vi "testAssertConnectorPanesMatchExpectedMissingFails.vi"(8 "error in (no error)":errorcluster, 11 "TestCase in":refnum<class "VeriStandTestCaseUnitTests.lvclass">) -> (0 "error out":errorcluster, 3 "TestCase out":refnum<class "VeriStandTestCaseUnitTests.lvclass">)   [LabVIEW 2015, in "VeriStandTestCaseUnitTests.lvclass"]
uses:
  VeriStandTestCaseUnitTests.lvclass
  <userlib>/_OpenG.lib/file/file.llb/Build Path - File Names Array - path__ogtk.vi
  <vilib>/addons/_JKI Toolkits/VI Tester/TestCase.llb/TestCase.lvclass
  VeriStandTestCase.lvclass
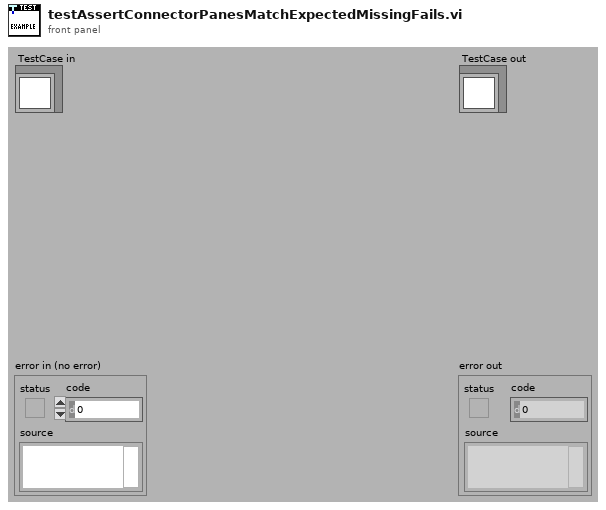
[diagram p1: front panel]
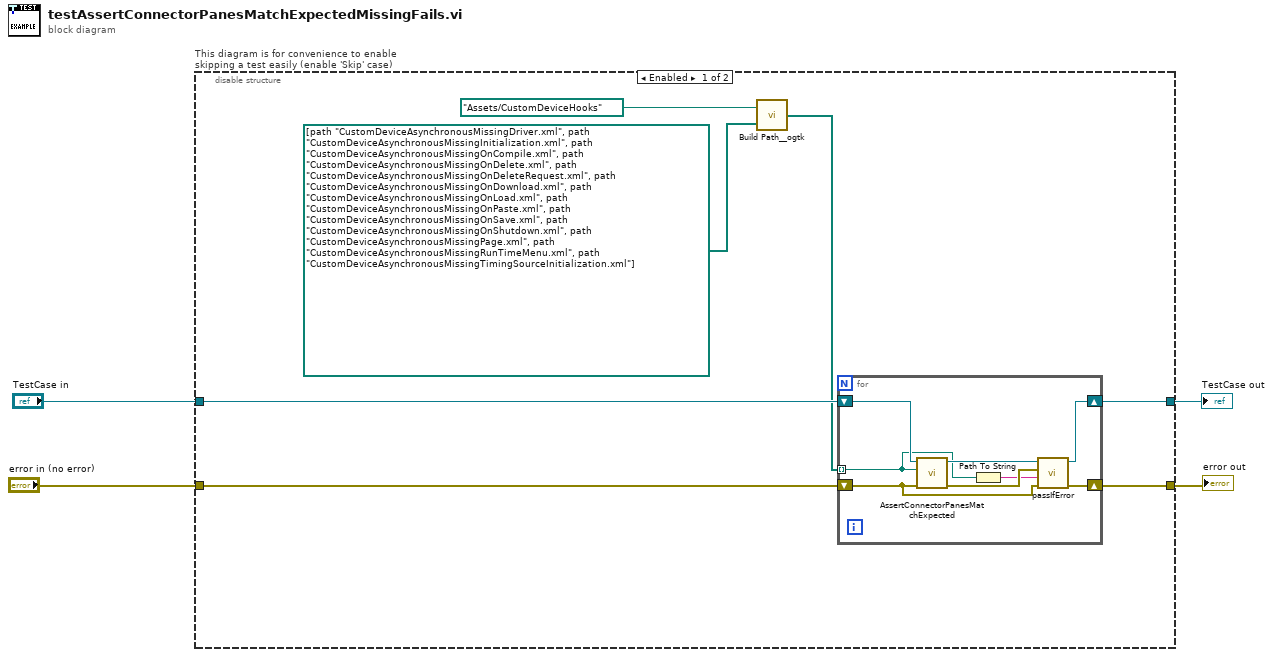
[diagram p0: block diagram]
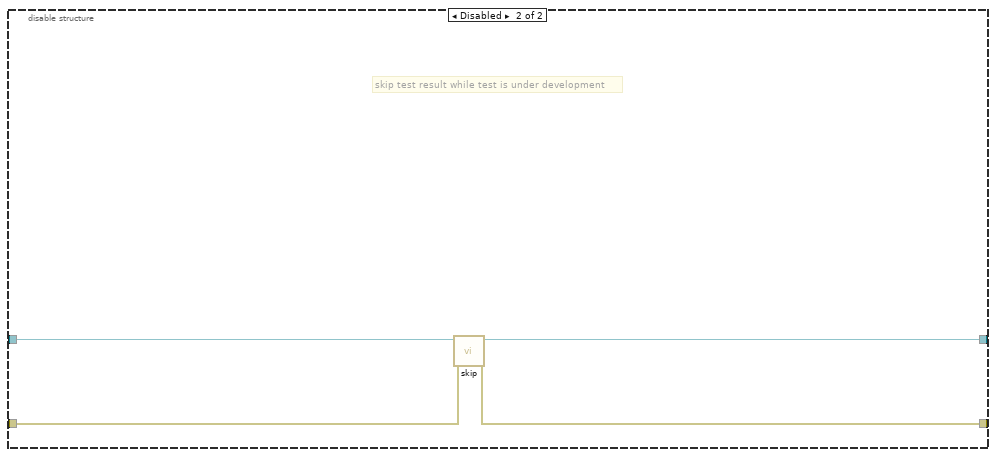
[diagram p2: hidden frame]
diagram:
  n1 = disable-structure "This diagram is for convenience to enable skipping a test easily (enable 'Skip' case)" shown="Enabled" {
    disable-tunnel: "TestCase in" -> [w9 w23]
    disable-tunnel: [w8 w21] -> w1
    disable-tunnel: [w10 w22] -> w3
    disable-tunnel: "error in (no error)" -> [w11 w20]
    frame Enabled {
      n2 = call-poly <userlib>:"Build Path__ogtk.vi"("name or relative path"=path[] [path "CustomDeviceAsynchronousMissingDriver.xml", path "CustomDeviceAsynchronousMissingInitialization.xml", path "CustomDeviceAsynchronousMissingOnCompile.xml", path "CustomDeviceAsynchronousMissingOnDelete.xml", path "CustomDeviceAsynchronousMissingOnDeleteRequest.xml", path "CustomDeviceAsynchronousMissingOnDownload.xml", path "CustomDeviceAsynchronousMissingOnLoad.xml", path "CustomDeviceAsynchronousMissingOnPaste.xml", path "CustomDeviceAsynchronousMissingOnSave.xml", path "CustomDeviceAsynchronousMissingOnShutdown.xml", path "CustomDeviceAsynchronousMissingPage.xml", path "CustomDeviceAsynchronousMissingRunTimeMenu.xml", path "CustomDeviceAsynchronousMissingTimingSourceInitialization.xml"], "base path"=path "Assets/CustomDeviceHooks") -> ("appended path"=w6:path[])
      n3 = for {
        tunnel: w6 -> [w13] mode=indexing
        shift-right: [w16] -> w10
        shift-left: w11 -> [w17]
        shift-right: [w14] -> w8
        shift-left: w9 -> [w15]
        n4 = call "AssertConnectorPanesMatchExpected.vi"("error in (no error)"=w17, "custom device xml path"=w13, "TestCase in"=w15) -> ("error out"=w18:errorcluster, "TestCase out"=w19:refnum<class "VeriStandTestCaseUnitTests.lvclass">)  [unwired: 7 in]
        n5 = Path To String(path=w13) -> (string=w12:string)
        n6 = call-dynamic "passIfError.vi"("error in (no error)"=w17, "task (\"\")"=w12, "error"=w18, "TestCase in"=w19) -> ("error out"=w16:errorcluster, "TestCase out"=w14:refnum<class "VeriStandTestCaseUnitTests.lvclass">)  [unwired: 6 in]
      }
    }
    frame Disabled {
      # "skip test result while test is under development"
      n7 = call <vilib>:"skip.vi"("error in (no error)"=w20, "TestCase in"=w23) -> ("error out"=w22:errorcluster, "TestCase out"=w21:refnum<class "VeriStandTestCaseUnitTests.lvclass">)  [unwired: 8 in]
    }
  }
  "error out" <- w3
  "TestCase out" <- w1
